vi "SetVelocity.vi"(8 "error in":errorcluster, 9 "Velocity":dbl, 11 "VISA resource":refnum<visa-resource-name>) -> (0 "error out":errorcluster)   [LabVIEW 2014, in "GRBLMotionCore.lvlib"]
uses:
  <instrlib>/GRBL/GRBLMotionCore.lvlib
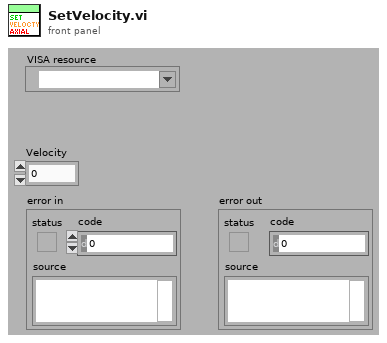
[diagram p1: front panel]
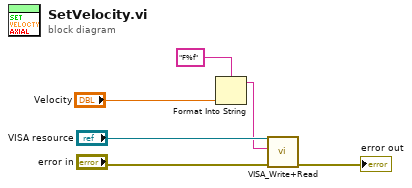
[diagram p0: block diagram]
diagram:
  n1 = Format Into String(format string="F%f", "Velocity") -> (resulting string=w2:string)  [unwired: 2 in, 1 out]
  n2 = call <instrlib>:"VISA_Write+Read.vi"("error in (no error)"="error in", "Write Buffer"=w2, "VISA resource name"="VISA resource") -> ("error out"=→"error out":errorcluster)  [unwired: 6 in, 2 out]
